vi "Pre Launch Init.vi"(11 "CANopen Test UI in":refnum<class "CANopen Test UI Actor.lvclass">) -> (0 "error out":errorcluster, 3 "CANopen Test UI out":refnum<class "CANopen Test UI Actor.lvclass">)   [LabVIEW 2024, in "CANopen Test UI Actor.lvlib" / "CANopen Test UI Actor.lvclass"]
doc: "<p>(<strong>Filename</strong>: <span class=\"dnl\">Actor Framework.lvlib:Actor.lvclass:Pre Launch Init.vi</span>)</p>\n<p>Defines behavior that occurs after the <a href=\"nihelplauncher://docs/csh?context=lvcore_lvcomm_af_launch_nested_actor\">Launch Nested Actor</a> method is invoked but before the actor's Actor Core method begins running.</p>\n<p>By default, this method does nothing. A descendant class may override it to define behavior.</p>"
uses:
  CANopen Test UI Actor.lvclass
  CANopen Test UI Actor.lvclass/CANopen Test UI Actor.ctl
  <vilib>/ActorFramework/Actor/Actor.lvclass
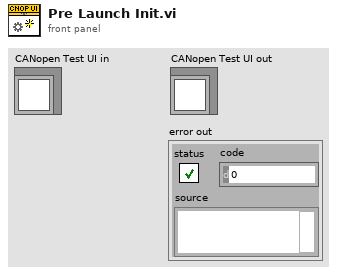
[diagram p1: front panel]
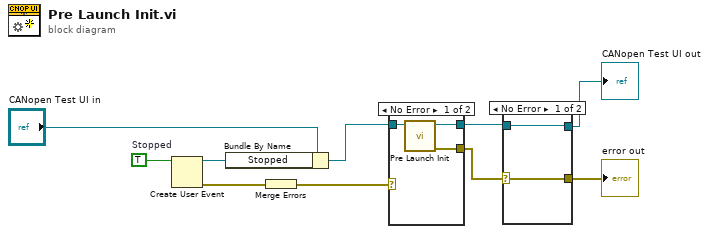
[diagram p0: block diagram]
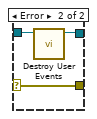
[diagram p3: hidden frame]
diagram:
  w10 = TRUE  # Stopped
  n1 = Create User Event(user event datatype=w10) -> (user event=w8:refnum<user-event>, error out=w7:errorcluster)  [unwired: 1 in]
  n2 = Bundle By Name(cluster="CANopen Test UI in", "Stopped"=w8) -> (w3:refnum<class "CANopen Test UI Actor.lvclass">)
  n3 = Merge Errors(w7) -> (w4:errorcluster)
  n4 = case shown="No Error" w4 {
    selector: w4 -> [_ w15]
    tunnel: [w13 w15] -> w2
    tunnel: [w12 w14] -> w6
    tunnel: w3 -> [w11 w14]
    frame No Error {
      n5 = call-parent "Pre Launch Init.vi"("Actor in"=w11) -> ("error out"=w13:errorcluster, "Actor out"=w12:refnum<class "CANopen Test UI Actor.lvclass">)  [unwired: 9 in]
    }
    frame Error {
    }
  }
  n6 = case shown="No Error" w2 {
    selector: w2 -> [w16 w18]
    tunnel: [w17 w20] -> w5
    tunnel: w6 -> [w17 w19]
    tunnel: [w16 w18] -> w1
    frame No Error {
    }
    frame Error {
      n7 = call "Destroy User Events.vi"("CANopen Test UI in"=w19) -> ("CANopen Test UI out"=w20:refnum<class "CANopen Test UI Actor.lvclass">)  [unwired: 10 in]
    }
  }
  "error out" <- w1
  "CANopen Test UI out" <- w5
